vi "Initialize.vi"(0 "VISA IN":refnum<visa-resource-name>, 1 "ID Query? (T: Yes)":bool=TRUE, 2 "Reset? (T: Yes)":bool=TRUE, 5 "error in":errorcluster) -> (14 "VISA Out":refnum<visa-resource-name>, 16 "Response":string, 19 "error out":errorcluster)   [LabVIEW 2018, in "PNA-X.lvlib"]
uses:
  PNA-X.lvlib
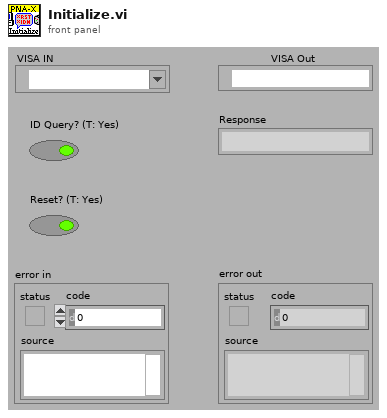
[diagram p1: front panel]
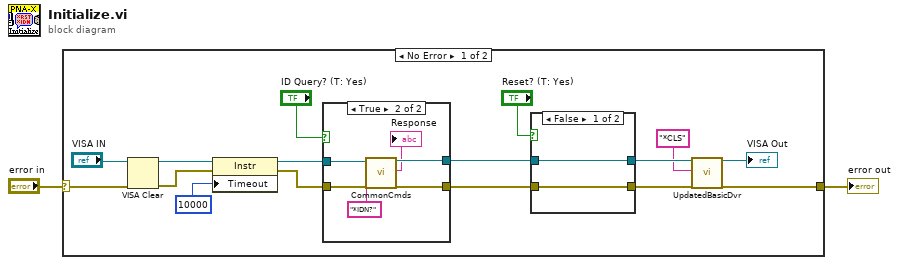
[diagram p0: block diagram]
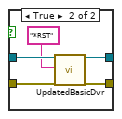
[diagram p3: hidden frame]
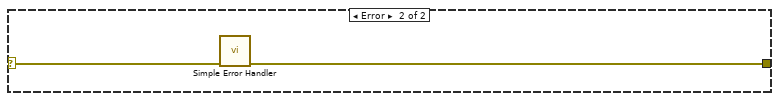
[diagram p4: hidden frame]
diagram:
  n1 = case shown="No Error" "error in" {
    selector: "error in" -> [w13 w35]
    tunnel: [w3 w34] -> w2
    frame No Error {
      n2 = VISA Clear(VISA resource name="VISA IN", error in (no error)=w13) -> (VISA resource name out=w11:refnum<visa-resource-name>, error out=w9:errorcluster)
      n3 = property class="Instr"(reference=w11, error in=w9, "Timeout"=u32 10000 ("General Settings:Timeout Value")) -> (reference out=w10:refnum<visa-resource-name>, error out=w8:errorcluster)
      n4 = case shown="True" "ID Query? (T: Yes)" {
        tunnel: [w19 w26] -> w18
        tunnel: [w20 w25] -> w16
        tunnel: w10 -> [w20 w24]
        tunnel: w8 -> [w19 w23]
        frame False {
        }
        frame True {
          n5 = call "CommonCmds.vi"("VISA IN"=w24, "error in"=w23, "Cmds"="*IDN?") -> ("VISA Out"=w25:refnum<visa-resource-name>, "Response"=→"Response":string, "error out"=w26:errorcluster)  [unwired: 14 in]
        }
      }
      n6 = case shown="False" "Reset? (T: Yes)" {
        tunnel: w18 -> [w27 w33]
        tunnel: [w27 w32] -> w17
        tunnel: w16 -> [w28 w31]
        tunnel: [w28 w30] -> w15
        frame False {
        }
        frame True {
          n7 = call "UpdatedBasicDvr.vi"("VISA IN"=w31, "Cmdline"="*RST", "error in"=w33) -> ("VISA Out"=w30:refnum<visa-resource-name>, "error out"=w32:errorcluster)  [unwired: 15 in]
        }
      }
      n8 = call "UpdatedBasicDvr.vi"("VISA IN"=w15, "Cmdline"="*CLS", "error in"=w17) -> ("VISA Out"=→"VISA Out":refnum<visa-resource-name>, "error out"=w3:errorcluster)  [unwired: 15 in]
    }
    frame Error {
      n9 = call <vilib>:"Simple Error Handler.vi"("error in (no error)"=w35) -> ("error out"=w34:errorcluster)  [unwired: 4 in, 4 out]
    }
  }
  "error out" <- w2
